vi "Wait.vi"(8 "error in (no error)":errorcluster, 11 "Model in":refnum<class "Model.lvclass">) -> (0 "error out":errorcluster, 3 "Model out":refnum<class "Model.lvclass">)   [LabVIEW 2015, in "Model.lvclass"]
uses:
  Model.lvclass
  Model.lvclass/Model.ctl
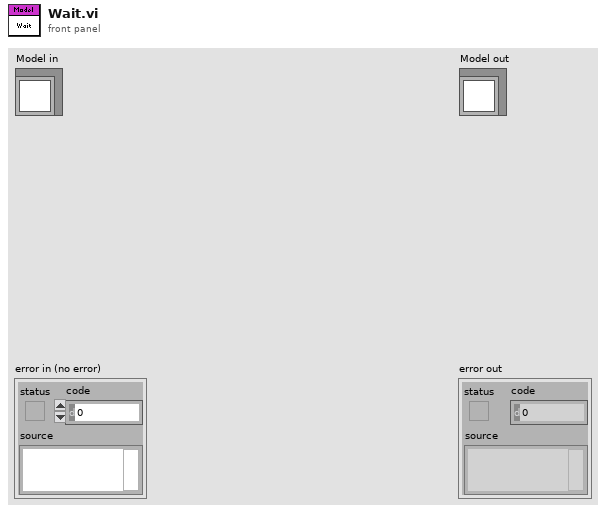
[diagram p1: front panel]
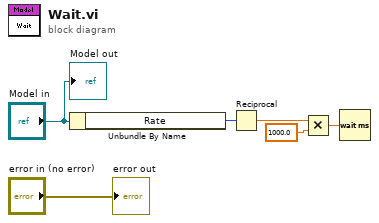
[diagram p0: block diagram]
diagram:
  n1 = Unbundle By Name("Model in") -> ("Rate"=w4:u8)
  n2 = Reciprocal(x=w4) -> (1/x=w3:dbl)
  n3 = Multiply(x=w3, y=1000.0) -> (x*y=w1:dbl)
  n4 = Wait (ms)(milliseconds to wait=w1) -> ()  [unwired: 1 out]
  "error out" <- "error in (no error)"
  "Model out" <- "Model in"
